vi "Configure AO task.vi"(8 "error in (no error)":errorcluster, 10 "analog generation":T1={"output rate"=0.0, "range"=0.0, "terminal configuration"=enum."Pseudodifferential", "output impedance"=0.0, "common mode offset"=0.0, "pure tone mode"=FALSE}, 11 "physical channels":tag) -> (0 "error out":errorcluster, 1 "number of channels":u32, 2 "actual sample rate":dbl, 3 "task out":refnum<k21>)   [LabVIEW 2021, in "AnalogGenerationProcess.lvlib"]
uses:
  AnalogGenerationProcess.lvlib
  controls/analog output settings.ctl
  controls/terminal configuration.ctl
  <vilib>/DAQmx/create/channels.llb/DAQmx Create Channel (AO-Voltage-Basic).vi
  <vilib>/DAQmx/configure/timing.llb/DAQmx Timing (Sample Clock).vi
  <resource>/objmgr/daqmx.rc
  controls/AudioGenTypeDefs.lvlib
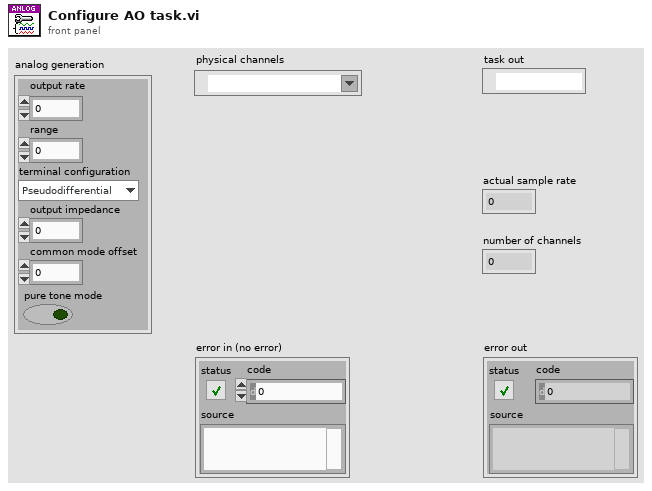
[diagram p1: front panel]
types:
  T1 = typedef "AudioGenTypeDefs.lvlib/analog output settings.ctl" = cluster{"output rate":dbl, "range":dbl, "terminal configuration":T2, "output impedance":dbl, "common mode offset":dbl, "pure tone mode":bool}
  T2 = typedef "AudioGenTypeDefs.lvlib/terminal configuration.ctl" = enum32{"Default", "RSE", "Differential", "Pseudodifferential"}
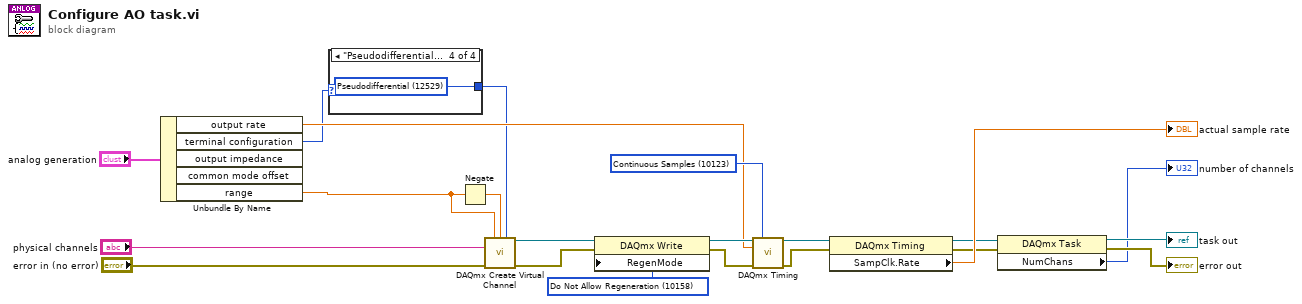
[diagram p0: block diagram]
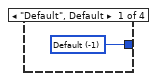
[diagram p2: hidden frame]
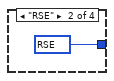
[diagram p3: hidden frame]
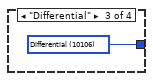
[diagram p4: hidden frame]
diagram:
  w14 = 10123 items=["Finite Samples"=10178, "Continuous Samples"=10123, "Hardware Timed Single Point"=12522] ("sample mode")
  w15 = 10158 items=["Allow Regeneration"=10097, "Do Not Allow Regeneration"=10158] ("RegenMode")
  n1 = Unbundle By Name("analog generation") -> ("output rate"=w10:dbl, "terminal configuration"=w6:T2, "range"=w9:dbl)  [unwired: 2 out]
  n2 = case shown="\"Pseudodifferential\"" w6 {
    tunnel: [w23 w24 w25 w26] -> w7
    frame "Default", Default {
      w23 = -1 items=["Default"=-1, "RSE"=10083, "Differential"=10106, "Pseudodifferential"=12529] ("output terminal configuration")
    }
    frame "RSE" {
      w24 = 10083 items=["Default"=-1, "RSE"=10083, "Differential"=10106, "Pseudodifferential"=12529] ("output terminal configuration")
    }
    frame "Differential" {
      w25 = 10106 items=["Default"=-1, "RSE"=10083, "Differential"=10106, "Pseudodifferential"=12529] ("output terminal configuration")
    }
    frame "Pseudodifferential" {
      w26 = 12529 items=["Default"=-1, "RSE"=10083, "Differential"=10106, "Pseudodifferential"=12529] ("output terminal configuration")
    }
  }
  n3 = Negate(x=w9) -> (-x=w13:dbl)
  n4 = call-poly <vilib>:"DAQmx Create Virtual Channel.vi"("maximum value"=w9, "minimum value"=w13, "output terminal configuration"=w7, "physical channels"="physical channels", "error in"="error in (no error)") -> ("task out"=w17:refnum<k21>, "error out"=w16:errorcluster)  [unwired: 9 in]
  n5 = property class="DAQmx Write"(reference=w17, error in=w16, "RegenMode"=w15) -> (reference out=w19:refnum<k21>, error out=w18:errorcluster)
  n6 = call-poly <vilib>:"DAQmx Timing.vi"("task/channels in"=w19, "sample mode"=w14, "rate"=w10, "error in"=w18) -> ("task out"=w21:refnum<k21>, "error out"=w20:errorcluster)  [unwired: 10 in]
  n7 = property class="DAQmx Timing"(reference=w21, error in=w20) -> (reference out=w5:refnum<k21>, error out=w4:errorcluster, "SampClk.Rate"=→"actual sample rate":dbl)
  n8 = property class="DAQmx Task"(reference=w5, error in=w4) -> (reference out=→"task out":refnum<k21>, error out=→"error out":errorcluster, "NumChans"=→"number of channels":u32)
